vi "Log Batteries.vi"(6 "BMS Low Voltage Status":T1 {"Temp. 0" scale=0.0..80.0; "Temp. 1" scale=0.0..80.0}, 7 "Battery Status":T2, 8 "BMS Status":T3, 9 "Log File Cluster":T4) -> ()   [LabVIEW 2016]
uses:
  Log File Cluster.ctl
  BMS Status.ctl
  RT/Battery Status.ctl
  RT/BMS Voltage status 2.ctl
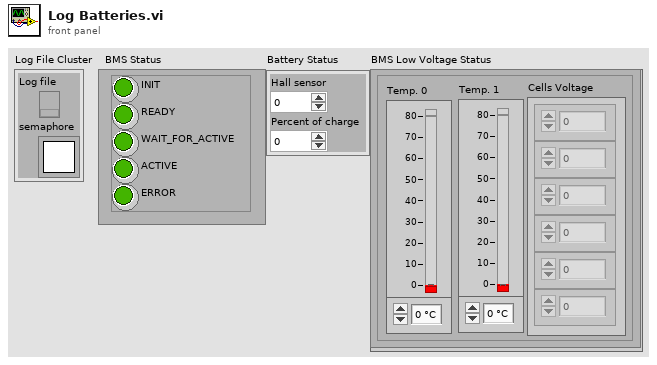
[diagram p1: front panel]
types:
  T1 = typedef "BMS Voltage status 2.ctl" = cluster{"Cells Voltage":dbl[], "Temp. 1":u8, "Temp. 0":u8}
  T2 = typedef "Battery Status.ctl" = cluster{"Hall sensor":i32, "Percent of charge":i16}
  T3 = typedef "BMS Status.ctl" = cluster{"INIT":bool, "READY":bool, "WAIT_FOR_ACTIVE":bool, "ACTIVE":bool, "ERROR":bool}
  T4 = typedef "Log File Cluster.ctl" = cluster{"Log file":refnum<k34>, "semaphore":T5}
  T5 = typedef "Semaphore RefNum" = refnum<k1>
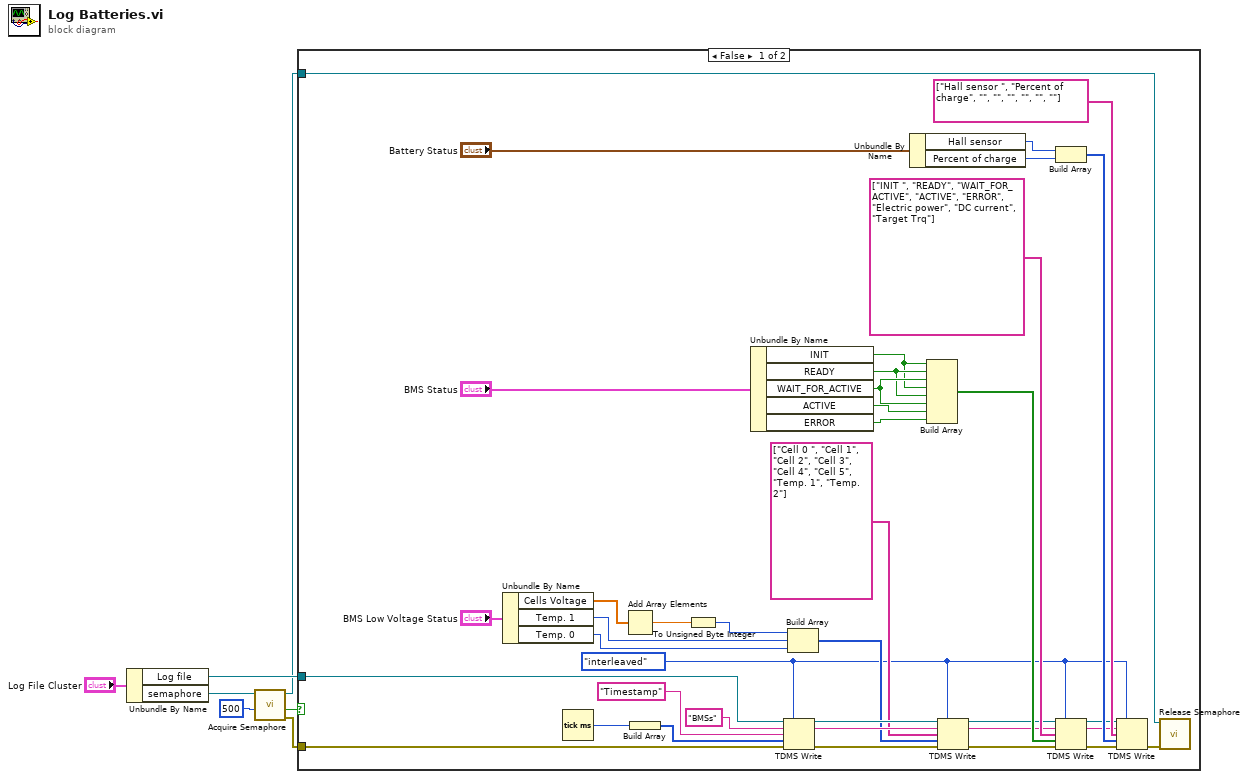
[diagram p0: block diagram]
diagram:
  n1 = Unbundle By Name("Log File Cluster") -> ("Log file"=w6:refnum<k34>, "semaphore"=w5:T5)
  n2 = call <vilib>:"Acquire Semaphore.vi"("ms timeout (-1)"=500, "semaphore"=w5) -> ("error out"=w4:errorcluster, "timed out"=w2:bool, "semaphore out"=w3:T5)  [unwired: 3 in]
  n3 = case shown="False" w2 {
    tunnel: w6 -> [w42 _]
    tunnel: w4 -> [w41 _]
    tunnel: w3 -> [w40 _]
    frame False {
      w11 = enum16{"decimated", "interleaved"}."interleaved" ("data layout (0:decimated)")
      n4 = Unbundle By Name("BMS Low Voltage Status") -> ("Cells Voltage"=w10:dbl[], "Temp. 1"=w37:u8, "Temp. 0"=w36:u8)
      n5 = Tick Count (ms)() -> (millisecond timer value=w46:u32)
      n6 = Add Array Elements(numeric array=w10) -> (sum=w8:dbl)
      n7 = Build Array(w46) -> (w45:u32[])
      n8 = To Unsigned Byte Integer(number=w8) -> (unsigned 8bit integer=w9:u8)
      n9 = Unbundle By Name("BMS Status") -> ("INIT"=w27:bool, "READY"=w28:bool, "WAIT_FOR_ACTIVE"=w29:bool, "ACTIVE"=w38:bool, "ERROR"=w39:bool)
      n10 = TDMS Write(0:w42, 1:w11, 5:"BMSs" ("group name in (Untitled)"), 7:"Timestamp", 9:w45, 11:w41) -> (4:w33:refnum<k34>, 6:w34:string, 15:w35:errorcluster)  [unwired: 1 out]
      n11 = Build Array(w9, w37, w36) -> (w24:u8[])
      n12 = Unbundle By Name("Battery Status") -> ("Hall sensor"=w26:i32, "Percent of charge"=w25:i16)
      n13 = Build Array(w27, w28, w29, w27, w28, w29, w38, w39) -> (w20:bool[])
      n14 = TDMS Write(0:w33, 1:w11, 5:w34, 7:string[] ["Cell 0 ", "Cell 1", "Cell 2", "Cell 3", "Cell 4", "Cell 5", "Temp. 1", "Temp. 2"] ("channel name(s) in (Untitled)"), 9:w24, 11:w35) -> (4:w14:refnum<k34>, 6:w15:string, 15:w22:errorcluster)  [unwired: 1 out]
      n15 = Build Array(w26, w25) -> (w18:i32[])
      n16 = TDMS Write(0:w14, 1:w11, 5:w15, 7:string[] ["INIT ", "READY", "WAIT_FOR_ACTIVE", "ACTIVE", "ERROR", "Electric power", "DC current", "Target Trq"] ("channel name(s) in (Untitled)"), 9:w20, 11:w22) -> (4:w13:refnum<k34>, 6:w16:string, 15:w21:errorcluster)  [unwired: 1 out]
      n17 = TDMS Write(0:w13, 1:w11, 5:w16, 7:string[] ["Hall sensor ", "Percent of charge", "", "", "", "", "", ""] ("channel name(s) in (Untitled)"), 9:w18, 11:w21) -> (15:w12:errorcluster)  [unwired: 3 out]
      n18 = call <vilib>:"Release Semaphore.vi"("error in (no error)"=w12, "semaphore"=w40) -> ()  [unwired: 4 in, 2 out]
    }
    frame True {
    }
  }
